vi "Untitled 8.vi"() -> ()   [LabVIEW 2021]
uses:
  Main/Ver_1/Config_File_Paths.ctl
panel:
  in  "Reset":bool
  out "Boolean":bool
  in  "Stop":bool
  in  "Measure":bool
  out "XY Graph":cluster{"Time":dbl[], "R":dbl[]}(graph)
  in  "Time unit":string(combo)="ms"
  in  "Config files paths":T1={"ZI config file (.ini)"="Config_Ver_1\\Zurich_params.ini", "Keithley config file (.ini)"="Config_Ver_1\\Keithley_params.ini", "Arduino config file (.ini)"="Config_Ver_1\\pulse_sequence.ini"}
  out "error out":errorcluster
  in  "Enum":T2(ring)=enum."Set Config"
  in  "Resource Address":T3={"ZI Address"="DEV714", "VISA Keithley"="", "VISA Arduino PG"=""}
  in  "error in":errorcluster
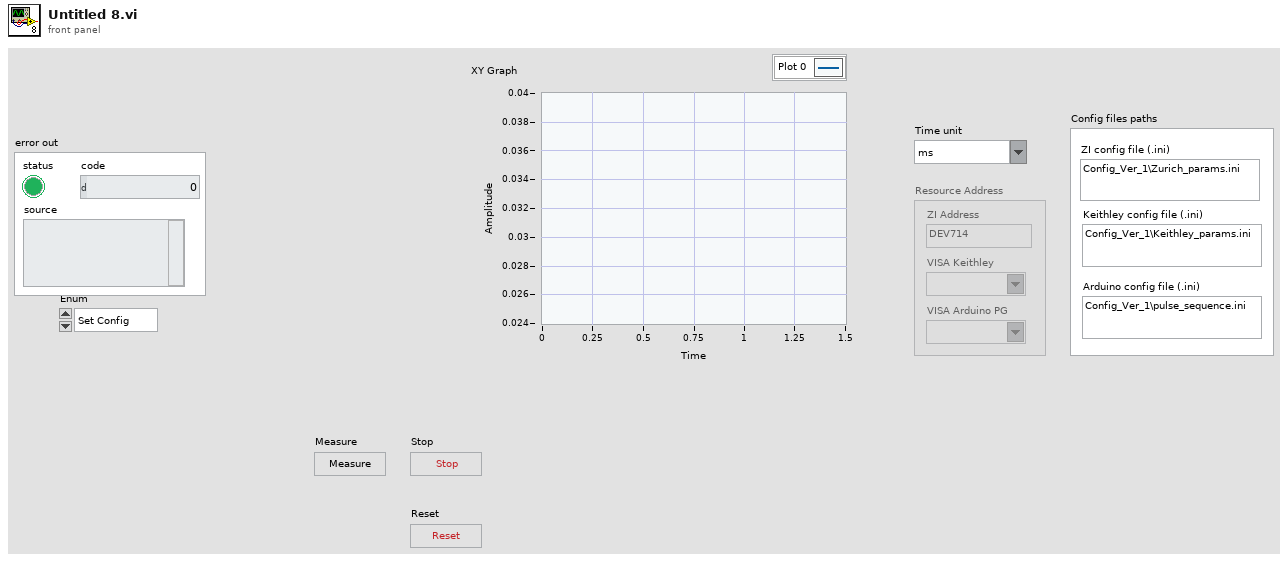
[diagram p1: front panel]
types:
  T1 = typedef "Config_File_Paths.ctl" = cluster{"ZI config file (.ini)":string, "Keithley config file (.ini)":string, "Arduino config file (.ini)":string}
  T2 = enum16{"Measurement average", "Close", "Wait", "Save", "Measurement", "Reset", "Set Config"}
  T3 = cluster{"ZI Address":string, "VISA Keithley":refnum<visa-resource-name>, "VISA Arduino PG":refnum<visa-resource-name>}
  T4 = enum8{"Enabled", "Disabled", "Disabled and Grayed Out"}
  T5 = typedef "Resources.ctl" = cluster{"ZI Handle":T6, "ZI ModHandle":T7, "VISA arduino":refnum<visa-resource-name>, "VISA Keithley":refnum<visa-resource-name>}
  T6 = typedef "Zurich Instruments LabOne.lvlib/ziTypeHandle.ctl" = cluster{"handleValid":bool, "Conn":u64, "Path Prefix":string, "Handle":u64, "Connected":bool, "Clockbase(s)":dbl}
  T7 = typedef "Zurich Instruments LabOne.lvlib/ziTypeModHandle.ctl" = cluster{"handleValid":bool, "Conn":u64, "ModHandle":u64, "moduleID":string, "Path Prefix":string}
  T8 = typedef "ZI_Data.ctl" = cluster{"R":dbl[], "Theta":dbl[], "X":dbl[], "Y":dbl[], "AuxIn1":dbl[], "AuxIn2":dbl[], "Frequency":dbl[], "DIO":dbl[], "Time":dbl[]}
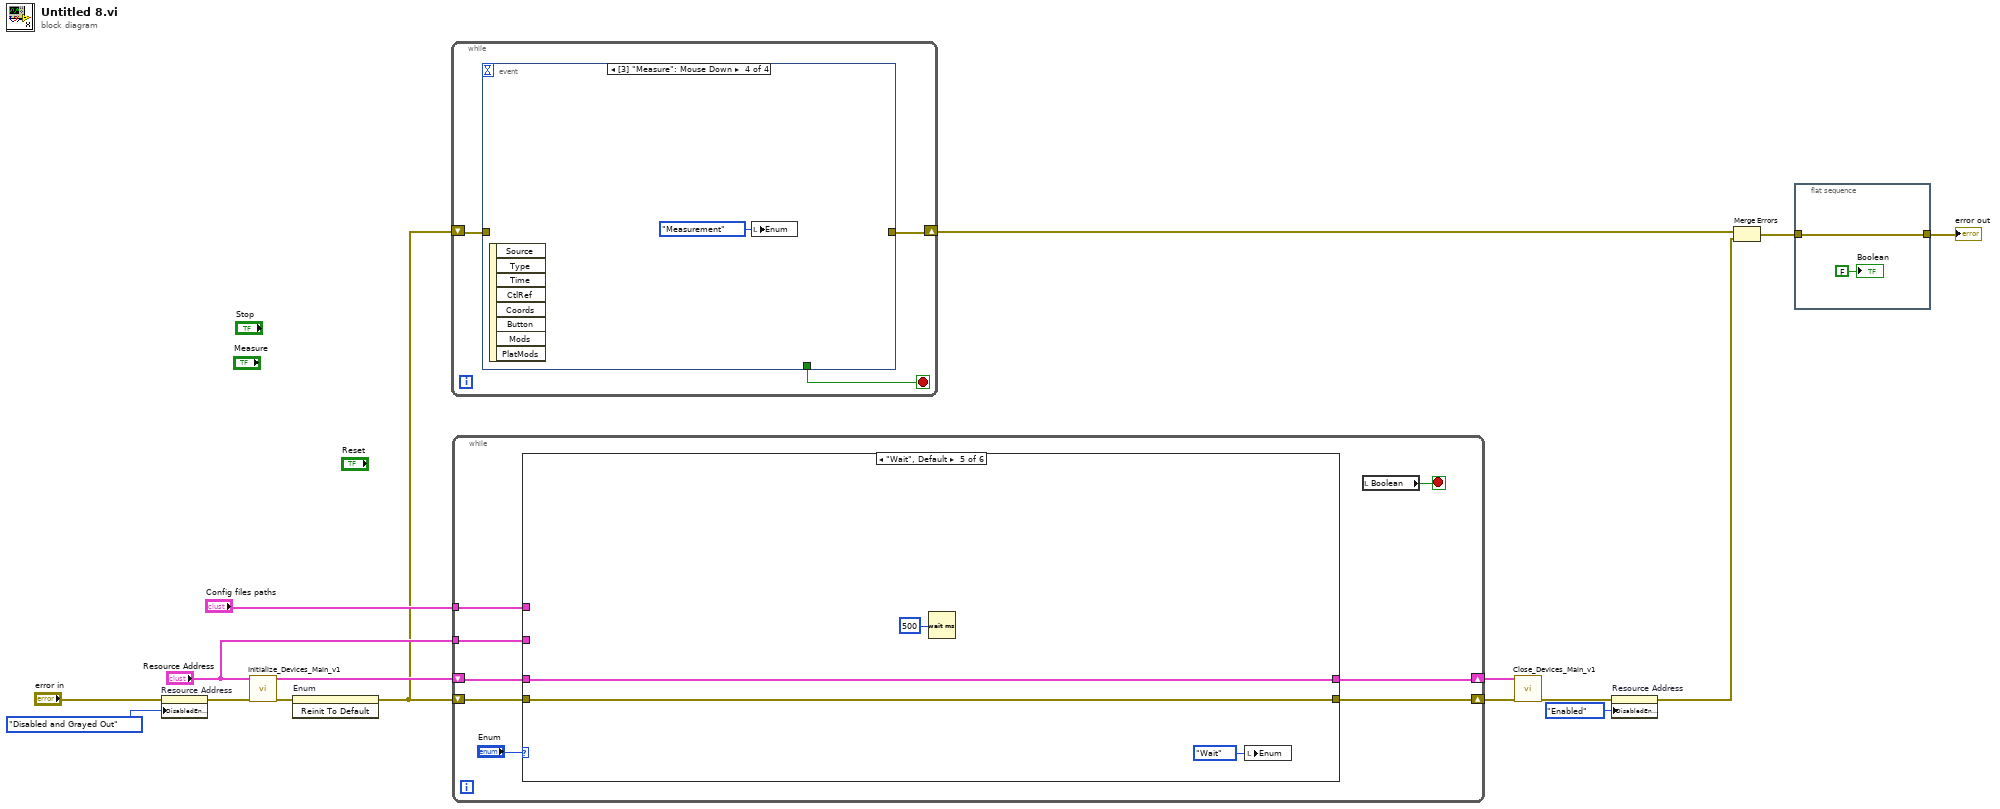
[diagram p0: block diagram]
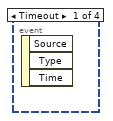
[diagram p2: hidden frame]
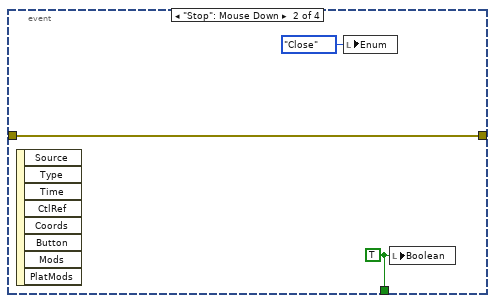
[diagram p3: hidden frame]
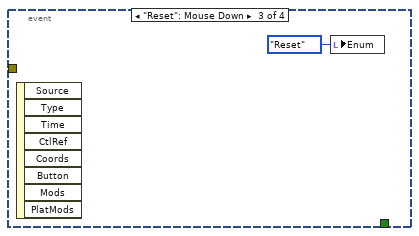
[diagram p4: hidden frame]
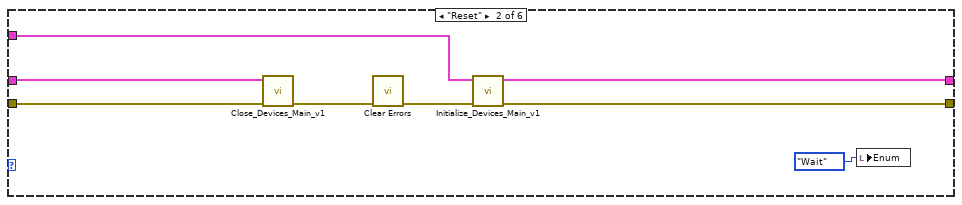
[diagram p6: hidden frame]
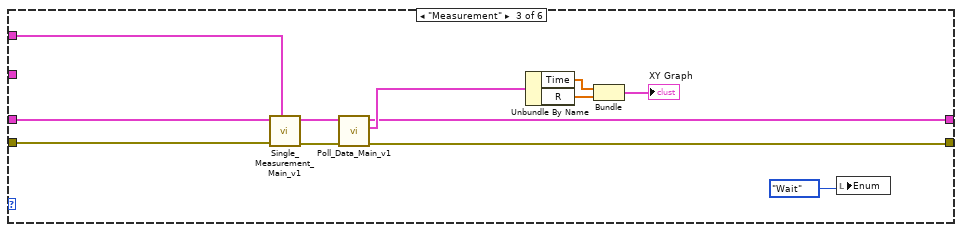
[diagram p7: hidden frame]
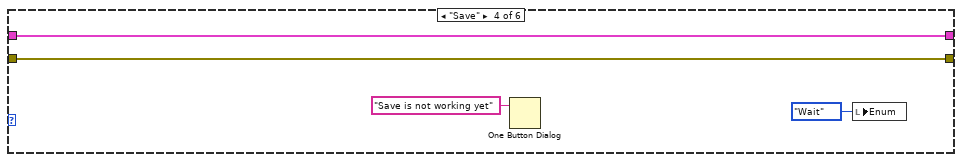
[diagram p8: hidden frame]
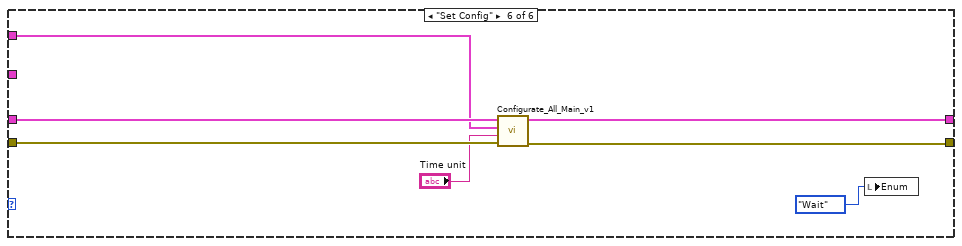
[diagram p9: hidden frame]
diagram:
  n1 = property on="Resource Address" class="Clust (strict)"(error in="error in", "DisabledEnum"=T4."Disabled and Grayed Out" ("Disabled")) -> (error out=w10:errorcluster)  [unwired: 1 in, 1 out]
  n2 = call "Initialize_Devices_Main_v1.vi"("error in"=w10, "Resource Address"="Resource Address") -> ("error out"=w2:errorcluster, "Resources"=w16:T5)  [unwired: 8 in]
  n3 = invoke on="Enum" class="Enum (strict)" method="Reinit To Default"(error in=w2) -> (error out=w1:errorcluster)  [unwired: 2 in, 2 out]
  n4 = while {
    shift-right: [w18] -> w6
    shift-left: w1 -> [w17]
    stop <- w19 stop-if-true
    n5 = event shown="[3] \"Measure\": Mouse Down" {
      selector: _ -> [_ _ _ _]
      dyn-events: _ -> [_ _ _ _]
      timeout: _ -> [_ _ _ _]
      tunnel: [_ w22 _ _] -> w19
      tunnel: [_ w21 _ _] -> w18
      tunnel: w17 -> [_ w21 _ _]
      event Timeout {
        n6 = event-data() -> ()  [unwired: 1 in, 3 out]
      }
      event "Stop": Mouse Down {
        w22 = TRUE ("Boolean")
        n7 = event-data() -> ()  [unwired: 1 in, 8 out]
        n8 = local write "Enum"(T2."Close" ("Enum")) -> ()
        n9 = local write "Boolean"(w22) -> ()
      }
      event "Reset": Mouse Down {
        n10 = event-data() -> ()  [unwired: 1 in, 8 out]
        n11 = local write "Enum"(T2."Reset" ("Enum")) -> ()
      }
      event "Measure": Mouse Down {
        n12 = event-data() -> ()  [unwired: 1 in, 8 out]
        n13 = local write "Enum"(T2."Measurement" ("Enum")) -> ()
      }
    }
  }
  n14 = while {
    shift-right: [w32] -> w15
    shift-left: w16 -> [w31]
    shift-right: [w30] -> w14
    shift-left: w1 -> [w29]
    tunnel: "Resource Address" -> [w28]
    tunnel: "Config files paths" -> [w27]
    stop <- w26 stop-if-true
    n15 = case shown="\"Wait\", Default" "Enum" {
      tunnel: [w34 w36 w45 w58 w62 w67] -> w32
      tunnel: w31 -> [w34 w38 w49 w58 w62 w69]
      tunnel: [w33 w39 w46 w57 w61 w66] -> w30
      tunnel: w29 -> [w33 w40 w48 w57 w61 w68]
      tunnel: w28 -> [_ w37 _ _ _ _]
      tunnel: w27 -> [_ _ w44 _ _ w64]
      frame "Close" {
      }
      frame "Reset" {
        n16 = call "Close_Devices_Main_v1.vi"("error in"=w40, "Resources in"=w38) -> ("error out"=w42:errorcluster)  [unwired: 9 in]
        n17 = call <vilib>:"Clear Errors.vi"("error in (no error)"=w42) -> ("error out"=w41:errorcluster)  [unwired: 5 in, 1 out]
        n18 = call "Initialize_Devices_Main_v1.vi"("error in"=w41, "Resource Address"=w37) -> ("error out"=w39:errorcluster, "Resources"=w36:T5)  [unwired: 8 in]
        n19 = local write "Enum"(T2."Wait" ("Enum")) -> ()
      }
      frame "Measurement" {
        n20 = call "Single_Measurement_Main_v1.vi"("Config files paths"=w44, "error in"=w48, "Resources In"=w49) -> ("error out"=w47:errorcluster, "Resources Out"=w50:T5)  [unwired: 7 in]
        n21 = call "Poll_Data_Main_v1.vi"("error in"=w47, "Resources in"=w50) -> ("error out"=w46:errorcluster, "ZI Data"=w52:T8, "Resources out"=w45:T5)  [unwired: 7 in]
        n22 = Unbundle By Name(w52) -> ("Time"=w51:dbl[], "R"=w53:dbl[])
        n23 = Bundle("Time"=w51, "R"=w53) -> (→"XY Graph":cluster{"Time":dbl[], "R":dbl[]})  [unwired: 1 in]
        n24 = local write "Enum"(T2."Wait" ("Enum")) -> ()
      }
      frame "Save" {
        n25 = One Button Dialog(message="Save is not working yet") -> ()  [unwired: 1 in, 1 out]
        n26 = local write "Enum"(T2."Wait" ("Enum")) -> ()
      }
      frame "Wait", Default {
        n27 = Wait (ms)(milliseconds to wait=u32 500) -> ()  [unwired: 1 out]
        n28 = local write "Enum"(T2."Wait" ("Enum")) -> ()
      }
      frame "Set Config" {
        n29 = call "Configurate_All_Main_v1.vi"("error in"=w68, "Time unit"="Time unit", "Config files paths"=w64, "Resources in"=w69) -> ("error out"=w66:errorcluster, "Resources out"=w67:T5)  [unwired: 4 in, 2 out]
        n30 = local write "Enum"(T2."Wait" ("Enum")) -> ()
      }
    }
    n31 = local read "Boolean"() -> (w26:bool)
  }
  n32 = call "Close_Devices_Main_v1.vi"("error in"=w14, "Resources in"=w15) -> ("error out"=w12:errorcluster)  [unwired: 9 in]
  n33 = property on="Resource Address" class="Clust (strict)"(error in=w12, "DisabledEnum"=T4."Enabled" ("Disabled")) -> (error out=w5:errorcluster)  [unwired: 1 in, 1 out]
  n34 = Merge Errors(w6, w5) -> (w4:errorcluster)
  n35 = flat-sequence {
    tunnel: w4 -> [w71]
    tunnel: [w71] -> w3
    frame #0 {
      "Boolean" <- FALSE ("Boolean")
    }
  }
  "error out" <- w3
